vi "CSE360_Final_Lab_Project.vi"() -> ()   [LabVIEW 2020]
panel:
  out "Motion":dbl(slide) scale=0.0..1.0
  out "Inches":dbl(knob) scale=0.0..50.0
  in  "Port 1":refnum<visa-resource-name>
  in  "Table":string[][](table)
  out "Inches":dbl(graph)
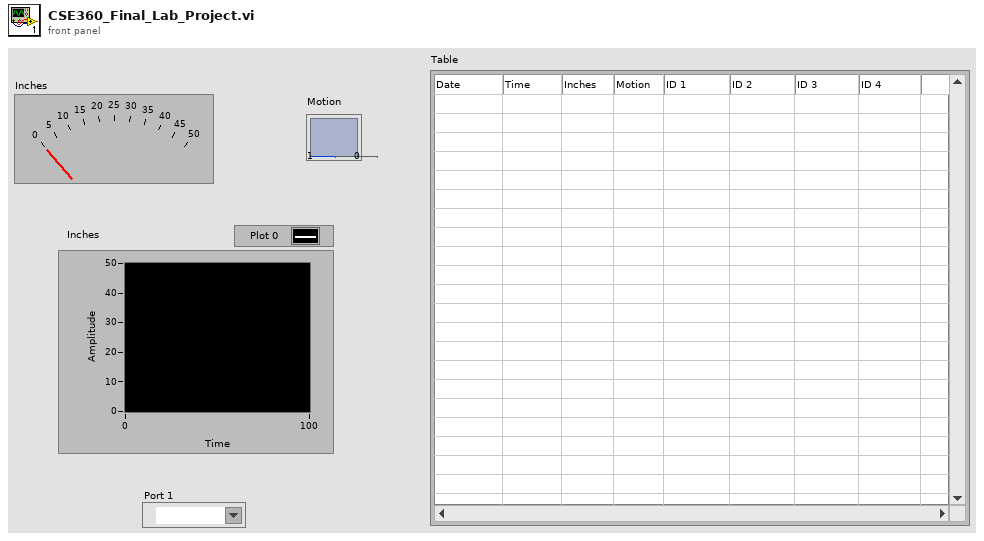
[diagram p1: front panel]
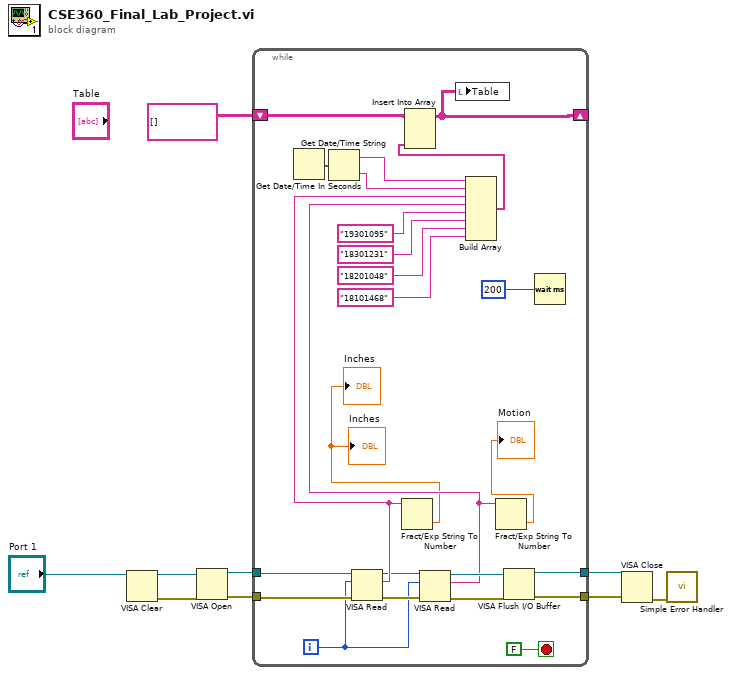
[diagram p0: block diagram]
diagram:
  n1 = VISA Clear(VISA resource name="Port 1") -> (VISA resource name out=w9:refnum<visa-resource-name>, error out=w8:errorcluster)  [unwired: 1 in]
  n2 = VISA Open(error in (no error)=w8, VISA resource name=w9) -> (VISA resource name=w6:refnum<visa-resource-name>, error out=w5:errorcluster)  [unwired: 3 in]
  n3 = while {
    tunnel: w6 -> [w34]
    tunnel: w5 -> [w33]
    tunnel: [w32] -> w4
    tunnel: [w31] -> w3
    shift-right: [w29] -> _
    shift-left: string[][] [] -> [w30]
    i -> [w18]
    stop <- FALSE stop-if-true
    n4 = Get Date/Time In Seconds() -> (seconds since 1Jan1904=w28:timestamp)
    n5 = Get Date/Time String(seconds (now)=w28) -> (date string=w27:string, time string=w26:string)  [unwired: 2 in]
    n6 = VISA Read(VISA resource name=w34, byte count=w18, error in (no error)=w33) -> (VISA resource name out=w22:refnum<visa-resource-name>, read buffer=w25:string, error out=w21:errorcluster)  [unwired: 1 out]
    n7 = Fract/Exp String To Number(string=w25) -> (number=→"Inches" →"Inches":dbl)  [unwired: 3 in, 1 out]
    n8 = VISA Read(VISA resource name=w22, byte count=w18, error in (no error)=w21) -> (VISA resource name out=w20:refnum<visa-resource-name>, read buffer=w17:string, error out=w19:errorcluster)  [unwired: 1 out]
    n9 = Build Array(w27, w26, w25, w17, "19301095" ("element"), "18301231" ("element"), "18201048" ("element"), "18101468" ("element")) -> (w23:string[])
    n10 = Insert Into Array(array=w30, new element=w23) -> (w29:string[][])  [unwired: 2 in]
    n11 = local write "Table"(w29) -> ()
    n12 = Fract/Exp String To Number(string=w17) -> (number=→"Motion":dbl)  [unwired: 3 in, 1 out]
    n13 = VISA Flush I/O Buffer(VISA resource name=w20, error in (no error)=w19) -> (VISA resource name out=w32:refnum<visa-resource-name>, error out=w31:errorcluster)  [unwired: 1 in]
    n14 = Wait (ms)(milliseconds to wait=u32 200) -> ()  [unwired: 1 out]
  }
  n15 = VISA Close(VISA resource name=w4, error in (no error)=w3) -> (error out=w7:errorcluster)
  n16 = call <vilib>:"Simple Error Handler.vi"("error in (no error)"=w7) -> ()  [unwired: 4 in, 5 out]
